vi "DSF.Engine.Memory.ObjectPool.Create.vi"(8 "error in (no error)":errorcluster, 11 "Objects":refnum<class>[](array[class])) -> (0 "error out":errorcluster, 3 "ObjectPool":refnum<class "DSF.Engine.Memory.ObjectPool.lvclass">)   [LabVIEW 2016, in "DSF.Engine.lvlib" / "DSF.Engine.Memory.ObjectPool.lvclass"]
uses:
  DSF.Engine.Memory.ObjectPool.lvclass
  DSF.Engine.Memory.ObjectPool.lvclass/DSF.Engine.Memory.ObjectPool.ctl
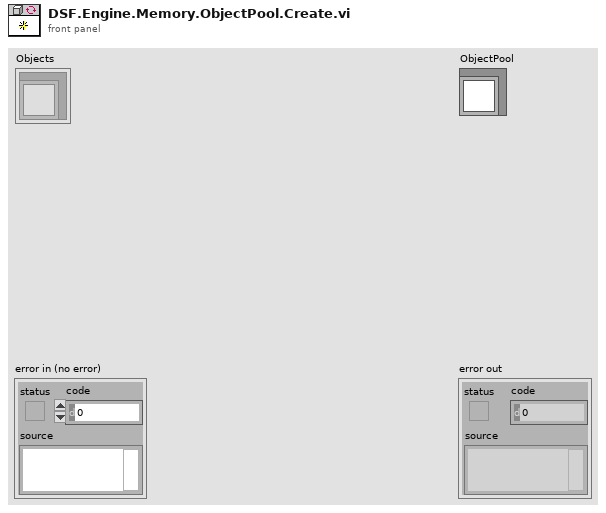
[diagram p1: front panel]
types:
  T1 = cluster{"read mode":enum16{"polling", "blocking"}, "write mode":enum16{"polling", "blocking"}}
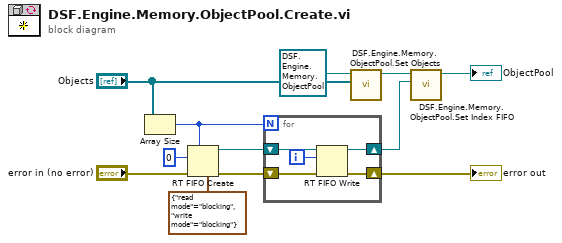
[diagram p0: block diagram]
diagram:
  n1 = Array Size(array="Objects") -> (size(s)=w5:i32)
  n2 = RT FIFO Create(1:0, 3:"error in (no error)", 4:w5, 7:T1 {"read mode"=enum."blocking", "write mode"=enum."blocking"} ("r/w modes (polling,polling)")) -> (8:w11:refnum<k33>, 11:w10:errorcluster)  [unwired: 4 in, 1 out]
  n3 = for {
    N: w5 -> [_]
    shift-right: [w15] -> w7
    shift-left: w10 -> [w13]
    shift-right: [w16] -> w2
    shift-left: w11 -> [w17]
    i -> [w14]
    n4 = RT FIFO Write(0:w17, 1:w14, 3:w13) -> (8:w16:refnum<k33>, 11:w15:errorcluster)  [unwired: 2 in, 2 out]
  }
  "error out" <- w7
  n5 = call "DSF.Engine.Memory.ObjectPool.Set Objects.vi"("Objects"="Objects", "ObjectPool in"=refnum<class "DSF.Engine.Memory.ObjectPool.lvclass"> refnum ("DSF.Engine.lvlib:ObjectPool")) -> ("ObjectPool out"=w3:refnum<class "DSF.Engine.Memory.ObjectPool.lvclass">)  [unwired: 8 in, 1 out]
  n6 = call "DSF.Engine.Memory.ObjectPool.Set Index FIFO.vi"("Index FIFO"=w2, "ObjectPool in"=w3) -> ("ObjectPool out"=→"ObjectPool":refnum<class "DSF.Engine.Memory.ObjectPool.lvclass">)  [unwired: 8 in, 1 out]
